vi "Get Selection.vi"(8 "error in (no error)":errorcluster, 10 "Wash":string, 11 "Attributes in":refnum<class "Attributes.lvclass">) -> (0 "error out":errorcluster, 3 "Attributes out":refnum<class "Attributes.lvclass">)   [LabVIEW 2021, in "Attributes.lvclass"]
uses:
  Attributes.lvclass
  Attributes.lvclass/Attributes.ctl
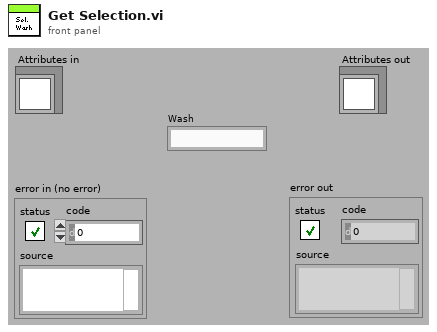
[diagram p1: front panel]
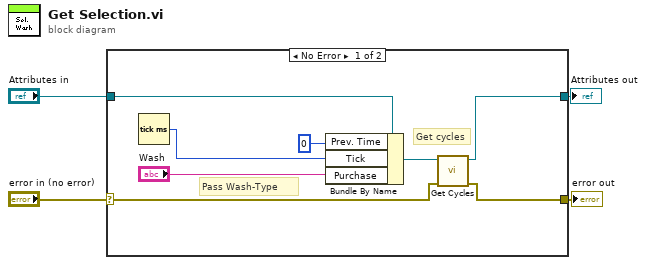
[diagram p0: block diagram]
diagram:
  n1 = case shown="No Error" "error in (no error)" {
    selector: "error in (no error)" -> [w10 w14]
    tunnel: [w9 w14] -> w3
    tunnel: [w7 w13] -> w1
    tunnel: "Attributes in" -> [w12 w13]
    frame No Error {
      # "Pass Wash-Type"
      # "Get cycles"
      n2 = Tick Count (ms)() -> (millisecond timer value=w6:u32)
      n3 = Bundle By Name(cluster=w12, "Prev. Time"=u32 0, "Tick"=w6, "Purchase"="Wash") -> (w8:refnum<class "Attributes.lvclass">)
      n4 = call-dynamic "Get Cycles.vi"("error in (no error)"=w10, "Attributes in"=w8) -> ("error out"=w9:errorcluster, "Attributes out"=w7:refnum<class "Attributes.lvclass">)  [unwired: 8 in]
    }
    frame Error {
    }
  }
  "error out" <- w3
  "Attributes out" <- w1
